vi "NI VeriStand - Open Project Reference.vi"(4 "Password":string, 6 "Username":string, 8 "error in (no error)":errorcluster, 10 "Gateway IP Address (\"\": localhost)":string, 11 "Project File Path":path) -> (0 "error out":errorcluster, 3 "Project Ref":T1)   [LabVIEW 2020, in "NI_VS Project ExecutionAPI.lvlib"]
doc: "Opens a reference to an NI VeriStand project."
uses:
  <vilib>/NI VeriStand/Execution/Project/NI_VS Project ExecutionAPI.lvlib
  <vilib>/NI VeriStand/Execution/Project/Project Ref.ctl
  NationalInstruments.VeriStand.ClientAPI
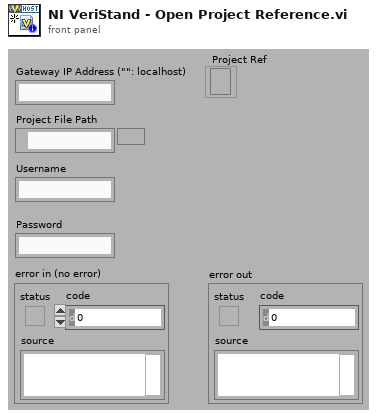
[diagram p1: front panel]
types:
  T1 = typedef "NI_VS Project ExecutionAPI.lvlib/Project Ref.ctl" = refnum<k24>
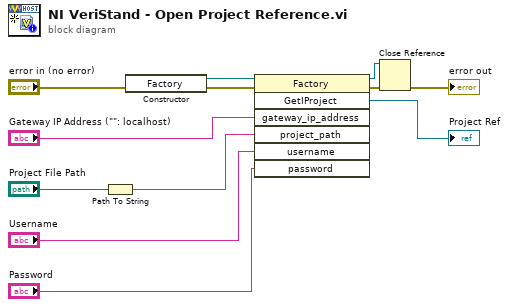
[diagram p0: block diagram]
diagram:
  n1 = Path To String(path="Project File Path") -> (string=w1:string)
  n2 = constructor class="Factory"(error in="error in (no error)") -> (reference out=w11:refnum<k24>, error out=w10:errorcluster)  [unwired: 2 in, 1 out]
  n3 = invoke class="Factory" method="GetIProject"(reference=w11, error in=w10, "gateway_ip_address"="Gateway IP Address (\"\": localhost)", "project_path"=w1, "username"="Username", "password"="Password") -> (reference out=w8:refnum<k24>, error out=w9:errorcluster, "GetIProject"=→"Project Ref":refnum<k24>)  [unwired: 1 in, 4 out]
  n4 = Close Reference(reference=w8, error in (no error)=w9) -> (error out=→"error out":errorcluster)
